vi "Create Execution Unit.vi"(8 "error in":errorcluster, 10 "Item Ref":T2=18446744073709551615 format="%.0x", 11 "Execution Unit Factory in":refnum<class "Execution Unit Factory.lvclass">) -> (0 "error out":errorcluster, 1 "Asynchronous Execution Units":T1[](array[typedef]) {"ReadWrite Channels" format="%.0x"; "Outgoing Channels" format="%.0x"; "Incoming Channels" format="%.0x"}, 2 "Inline Execution Units":T1[](array[typedef]) {"ReadWrite Channels" format="%.0x"; "Outgoing Channels" format="%.0x"; "Incoming Channels" format="%.0x"}, 3 "Execution Unit Factory out":refnum<class "Execution Unit Factory.lvclass">)   [LabVIEW 2020, in "AIM MIL-STD-1553 Engine.lvlib" / "Interfaces.lvlib" / "Execution Unit Factory.lvclass"]
uses:
  Execution Unit Factory.lvclass
  Controls/Execution Unit Information.ctl
  Execution Unit/Execution Unit.lvclass
  <vilib>/NI VeriStand/Custom Device API/Custom Device Item Ref.ctl
  <vilib>/NI VeriStand/Custom Device API/Custom Device API.lvlib
  Interfaces.lvlib
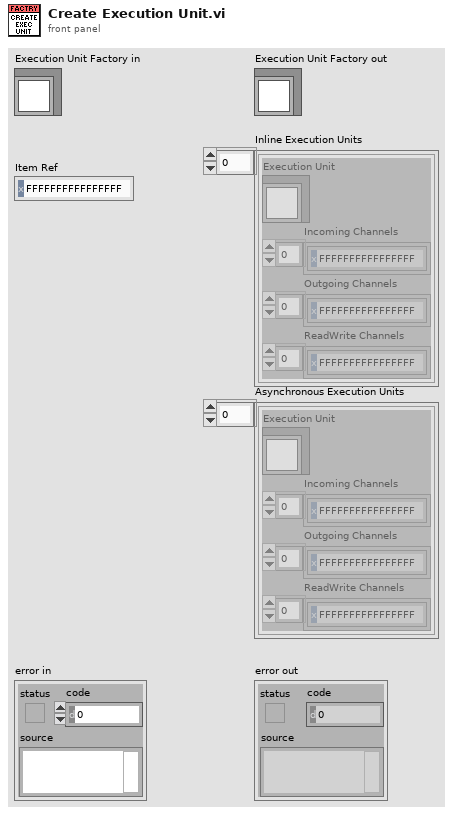
[diagram p1: front panel]
types:
  T1 = typedef "AIM MIL-STD-1553 Engine.lvlib/Interfaces.lvlib/Execution Unit Information.ctl" = cluster{"Execution Unit":refnum<class "Execution Unit.lvclass">, "Incoming Channels":T2[], "Outgoing Channels":T2[], "ReadWrite Channels":T2[]}
  T2 = typedef "Custom Device API.lvlib/Custom Device Item Ref.ctl" = u64
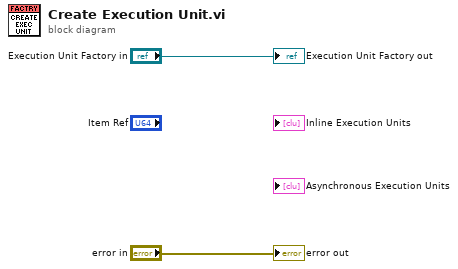
[diagram p0: block diagram]
diagram:
  "error out" <- "error in"
  "Execution Unit Factory out" <- "Execution Unit Factory in"
